vi "GET.vi"(6 "timeout (10000)":i32=10000, 7 "output file":path=path "", 8 "error in (no error)":errorcluster, 10 "url":string, 11 "HTTP Client Advanced in":refnum<class "HTTP Client Advanced.lvclass">) -> (0 "error out":errorcluster, 1 "body":string, 2 "headers":string, 3 "HTTP Client Advanced out":refnum<class "HTTP Client Advanced.lvclass">)   [LabVIEW 2021, in "HTTP Client Advanced.lvclass"]
uses:
  HTTP Client Advanced.lvclass
  HTTP Client Advanced.lvclass/HTTP Client Advanced.ctl
  <vilib>/NI/Advanced HTTP Client/Session.lvclass
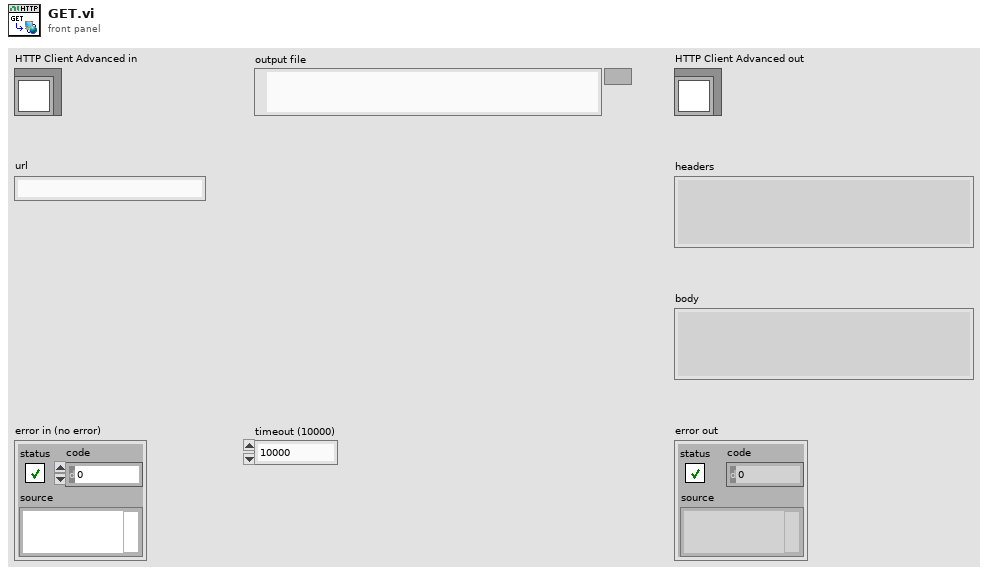
[diagram p1: front panel]
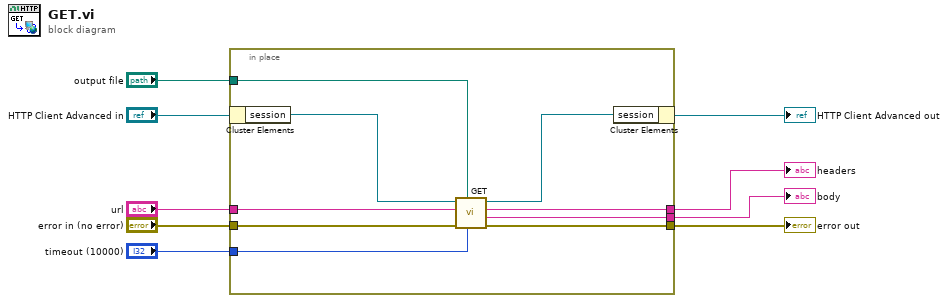
[diagram p0: block diagram]
diagram:
  n1 = in-place {
    in-place-border: [w17] -> w8
    in-place-border: "url" -> [w14]
    in-place-border: [w12] -> w3
    in-place-border: [w13] -> w4
    in-place-border: "error in (no error)" -> [w18]
    in-place-border: "output file" -> [w11]
    in-place-border: "timeout (10000)" -> [w10]
    n2 = in-place-cluster #1("HTTP Client Advanced in") -> ("session"=w16:refnum<class "Session.lvclass">)
    n3 = call <vilib>:"GET.vi"("timeout"=w10, "output file"=w11, "error in"=w18, "url"=w14, "session in"=w16) -> ("error out"=w17:errorcluster, "body"=w12:string, "headers"=w13:string, "session out"=w15:refnum<class "Session.lvclass">)  [unwired: 2 in, 1 out]
    n4 = in-place-cluster #1("session"=w15) -> (→"HTTP Client Advanced out":refnum<class "HTTP Client Advanced.lvclass">)
  }
  "error out" <- w8
  "headers" <- w4
  "body" <- w3
